vi "ReadWrite.ReadValues.vi"(8 "error in":errorcluster, 11 "ReadWrite in":refnum<class "ReadWrite.lvclass">) -> (0 "error out":errorcluster, 2 "Values":dbl[](array[numeric]), 3 "ReadWrite out":refnum<class "ReadWrite.lvclass">)   [LabVIEW 2024, in "VS Plugin Data Access Engine.lvlib" / "ReadWrite.lvclass"]
uses:
  ReadWrite.lvclass
  ReadWrite.lvclass/ReadWrite.ctl
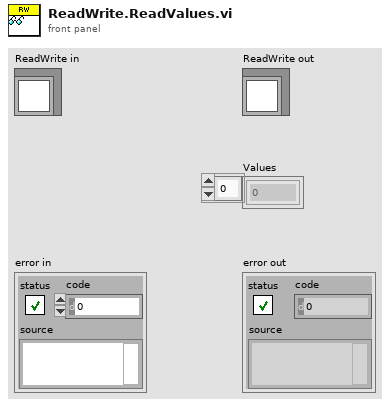
[diagram p1: front panel]
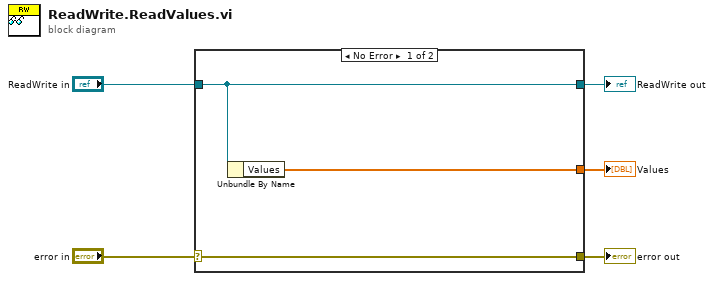
[diagram p0: block diagram]
diagram:
  n1 = case shown="No Error" "error in" {
    selector: "error in" -> [w8 w10]
    tunnel: [w8 w10] -> w4
    tunnel: [w7 w9] -> w2
    tunnel: "ReadWrite in" -> [w7 w9]
    tunnel: [w6 _] -> w1
    frame No Error {
      n2 = Unbundle By Name(w7) -> ("Values"=w6:dbl[])
    }
    frame Error {
    }
  }
  "error out" <- w4
  "ReadWrite out" <- w2
  "Values" <- w1
